vi "Write I-V parameters.vi"(8 "error in (no error)":errorcluster, 10 "I-V parameters":T1={"Start magnitude"=0.01, "Magnitude increment"=0.001, "Number of pulses"=8, "Baseline length"=0.00024576, "Ramp length"=1.6384e-05, "Top  length"=0.00024576, "Threshold "=1e-05} {"Threshold" format="%#_6p"; "Top  length" format="%#_6p"; "Ramp length" format="%#_6p"; "Baseline length" format="%#_6p"; "Magnitude increment" format="%#_6p"; "Start magnitude" format="%#_6p"}, 11 "RP I-V Driver in":refnum<class "RP I-V Driver.lvclass">) -> (0 "error out":errorcluster, 3 "RP I-V Driver out":refnum<class "RP I-V Driver.lvclass">)   [LabVIEW 2016, in "RP I-V Driver.lvclass"]
uses:
  RP I-V Driver.lvclass
  Waform generation/I-V parameters.ctl
  RP I-V Driver.lvclass/RP I-V Driver.ctl
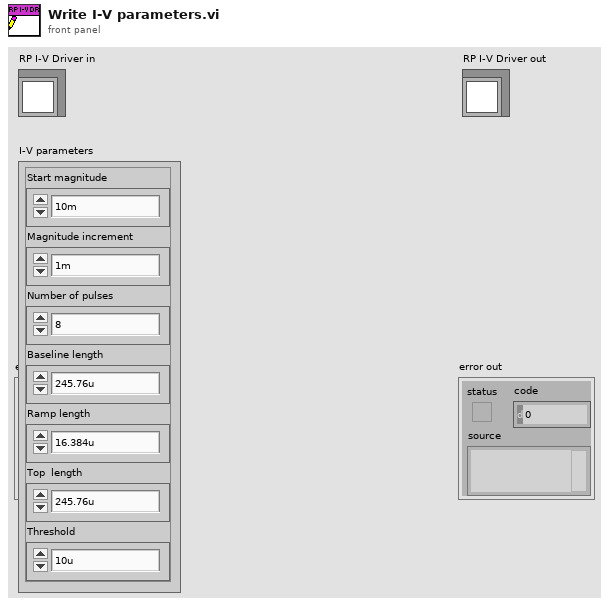
[diagram p1: front panel]
types:
  T1 = typedef "I-V parameters.ctl" = cluster{"Start magnitude":dbl, "Magnitude increment":dbl, "Number of pulses":i32, "Baseline length":dbl, "Ramp length":dbl, "Top  length":dbl, "Threshold ":dbl}
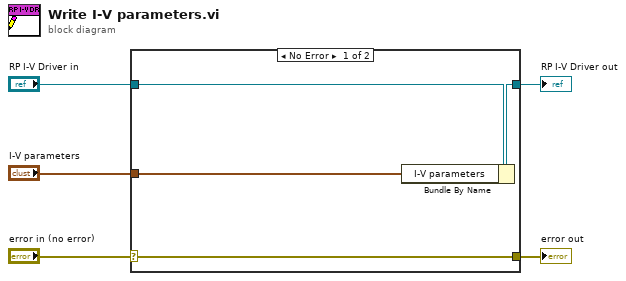
[diagram p0: block diagram]
diagram:
  n1 = case shown="No Error" "error in (no error)" {
    selector: "error in (no error)" -> [w9 w10]
    tunnel: [w9 w10] -> w4
    tunnel: [w7 w11] -> w2
    tunnel: "RP I-V Driver in" -> [w8 w11]
    tunnel: "I-V parameters" -> [w6 _]
    frame No Error {
      n2 = Bundle By Name(cluster=w8, "I-V parameters"=w6) -> (w7:refnum<class "RP I-V Driver.lvclass">)
    }
    frame Error {
    }
  }
  "error out" <- w4
  "RP I-V Driver out" <- w2
